vi "GroupInfo.vi"() -> ()   [LabVIEW 2014]
panel:
  out "group names":string[](array[string])
  out "error out":errorcluster
  in  "file path":path
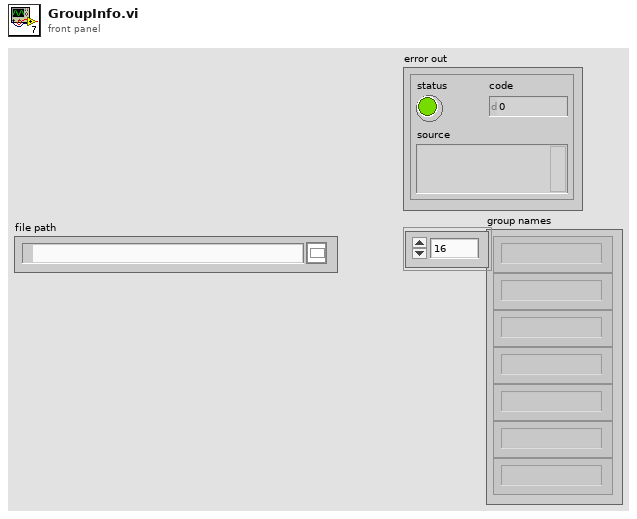
[diagram p1: front panel]
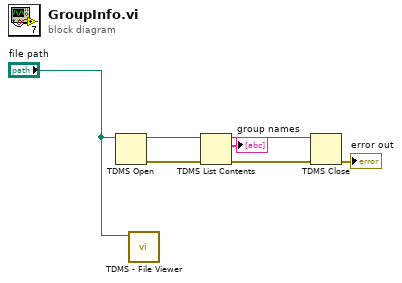
[diagram p0: block diagram]
diagram:
  n1 = TDMS Open(11:"file path") -> (0:w6:errorcluster, 3:w7:refnum<k34>)  [unwired: 6 in]
  n2 = call <vilib>:"TDMS - File Viewer.vi"("file path"="file path") -> ()  [unwired: 5 in, 2 out]
  n3 = TDMS List Contents(4:w6, 7:w7) -> (0:w5:errorcluster, 2:→"group names":string[], 3:w4:refnum<k34>)  [unwired: 1 in, 1 out]
  n4 = TDMS Close(8:w5, 11:w4) -> (0:→"error out":errorcluster)  [unwired: 1 out]
